vi "AddShooter.vi"(9 "Shooter Aligned":bool, 10 "Shooter Up":bool, 11 "Refnum in":T1) -> (3 "Refnum out":T1)   [LabVIEW 2019]
uses:
  <vilib>/vision/Image Controls.llb/IMAQ Image.ctl
  <vilib>/vision/NI_Vision_Development_Module.lvlib
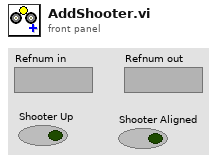
[diagram p1: front panel]
types:
  T1 = typedef "IMAQ Image.ctl" = refnum<image>
  T2 = typedef "Image Type" = u32
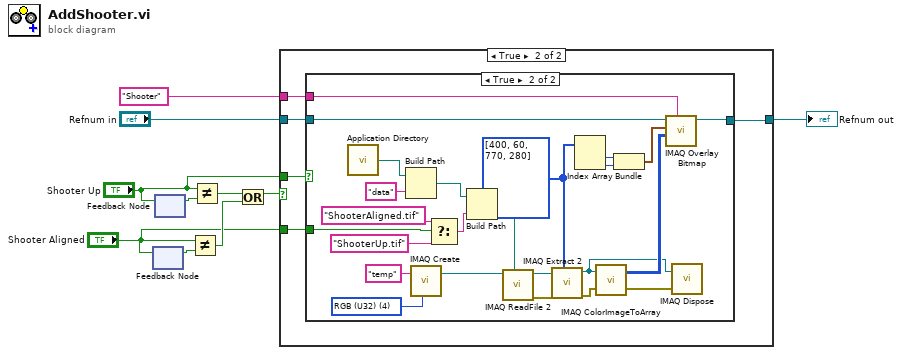
[diagram p0: block diagram]
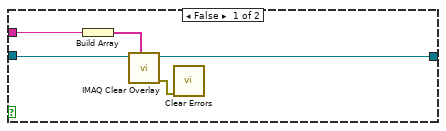
[diagram p3: hidden frame]
diagram:
  n1 = feedback #1() -> (w3:bool)  [unwired: 1 in]
  n2 = feedback-in #1("Shooter Aligned") -> ()
  n3 = feedback-in #2("Shooter Up") -> ()
  n4 = feedback #2() -> (w9:bool)  [unwired: 1 in]
  n5 = Not Equal?(x="Shooter Aligned", y=w3) -> (x != y?=w2:bool)
  n6 = Not Equal?(x="Shooter Up", y=w9) -> (x != y?=w10:bool)
  n7 = Or(x=w10, y=w2) -> (x .or. y?=w4:bool)
  n8 = case shown="True" w4 {
    tunnel: [w11 w14] -> w8
    tunnel: "Refnum in" -> [w11 w15]
    tunnel: "Shooter Up" -> [_ w16]
    tunnel: "Shooter" -> [_ w13]
    tunnel: "Shooter Aligned" -> [_ w12]
    frame False {
    }
    frame True {
      n9 = case shown="True" w16 {
        tunnel: w15 -> [w21 w44]
        tunnel: [w20 w43] -> w14
        tunnel: w13 -> [w19 w45]
        tunnel: w12 -> [_ w26]
        frame False {
          n10 = Build Array(w19) -> (w18:string[])
          n11 = call "IMAQ Clear Overlay"("Groups"=w18, "Image"=w21) -> ("error out"=w17:errorcluster, "Image Out"=w20:T1)  [unwired: 8 in]
          n12 = call <vilib>:"Clear Errors.vi"("error in (no error)"=w17) -> ()  [unwired: 5 in, 2 out]
        }
        frame True {
          w31 = i32[] [400, 60, 770, 280] ("Optional Rectangle")
          w37 = T2 4 items=["Grayscale (U8)", "Grayscale (I16)", "Grayscale (SGL)", "Complex (CSG)", "RGB (U32)", "HSL (U32)", "RGB (U64)", "Grayscale (U16)"] ("Image Type")
          n13 = call <vilib>:"Application Directory.vi"() -> ("Application Directory"=w41:path)
          n14 = Build Path(base path=w41, name or relative path="data") -> (appended path=w42:path)
          n15 = call "IMAQ Create"("Image Name"="temp", "Image Type"=w37) -> ("New Image"=w36:T1)  [unwired: 3 in, 1 out]
          n16 = Select(t="ShooterAligned.tif" ("name or relative path"), s=w26, f="ShooterUp.tif" ("name or relative path")) -> (s? t:f=w27:string)
          n17 = Build Path(base path=w42, name or relative path=w27) -> (appended path=w39:path)
          n18 = call "IMAQ ReadFile 2"("File Path"=w39, "Image"=w36) -> ("error out"=w35:errorcluster, "Image Out"=w34:T1)  [unwired: 5 in, 3 out]
          n19 = call "IMAQ Extract 2"("Optional Rectangle"=w31, "error in (no error)"=w35, "Image Src"=w34) -> ("error out"=w33:errorcluster, "Image Dst Out"=w22:T1)  [unwired: 7 in]
          n20 = Index Array(array=w31) -> (element #1=w29:i32, element #2=w30:i32)  [unwired: 2 in]
          n21 = call "IMAQ ColorImageToArray"("Image"=w22, "error in (no error)"=w33) -> ("Image Pixels (U32)"=w32:u32[][], "error out"=w23:errorcluster)  [unwired: 2 in, 1 out]
          n22 = Bundle(w29, w30) -> (w28:cluster{i32, i32})  [unwired: 1 in]
          n23 = call "IMAQ Overlay Bitmap"("Group"=w45, "Bitmap"=w32, "Top Left Point"=w28, "Image"=w44) -> ("Image Out"=w43:T1)  [unwired: 6 in, 1 out]
          n24 = call "IMAQ Dispose"("Image"=w22, "error in (no error)"=w23) -> ()  [unwired: 4 in, 1 out]
        }
      }
    }
  }
  "Refnum out" <- w8
